vi "Detector Set Config.vi"(8 "error in (no error)":errorcluster, 11 "RIMAS Detector in":refnum<class "RIMAS Detector.lvclass">) -> (0 "error out":errorcluster, 3 "RIMAS Detector out":refnum<class "RIMAS Detector.lvclass">)   [LabVIEW 2022 SP3, in "RIMAS Detector.lvclass"]
uses:
  RIMAS Detector.lvclass
  C:/Development/rimas/RIMAS/Detector/Detector Class/Detector Class.lvclass
  Detector Class.lvclass
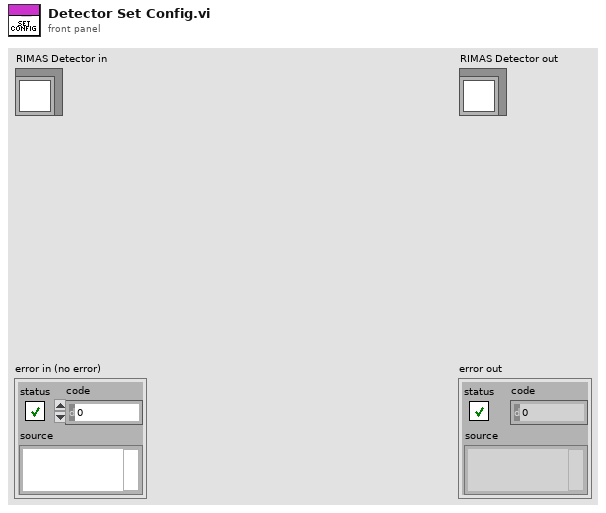
[diagram p1: front panel]
types:
  T1 = typedef "RIMAS Detector Config.ctl" = cluster{"Detector":u16, "Offsets":u16[][], "Detector Computer":T2, "FITS hdr template0":path, "FITS hdr template1":path, "FITS Data File Path":path, "FITS Detector Settings":T3, "Sim Folder":path, "Integration Mode":T4, "Integration Time":dbl, "Frame Int Time":dbl}
  T2 = typedef "RIMAS Detector Server Config.ctl" = cluster{"Machine":string, "Password":string, "FITS File Path":string, "Port":u16, "Header Path":string, "Name":string}
  T3 = typedef "RIMAS Observation Config.ctl" = cluster{"Exp Time Short":dbl, "# of Frames":dbl, "Exp Time Long":dbl, "# of Groups":dbl, "Object Name":string, "Object":string, "Obs Type":string, "Image Type":string, "Observer":string, "Observer Affiliation":string}
  T4 = typedef "Detector enum Detector Integration Mode.ctl" = enum16{"SSR", "CDS", "MEAN", "MEDIAN", "MODE", "MIIN", "MAX"}
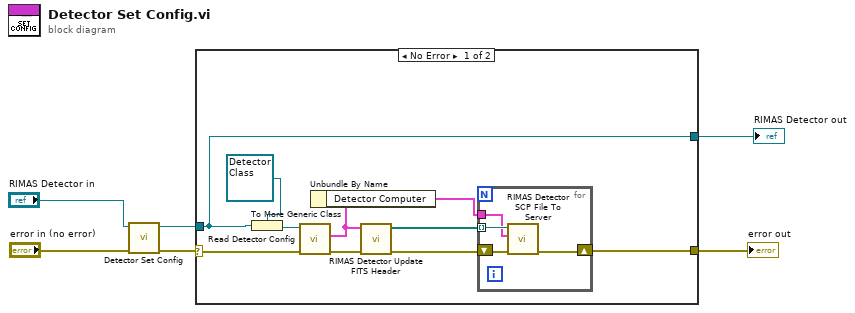
[diagram p0: block diagram]
diagram:
  n1 = call-parent "Detector Set Config.vi"("error in (no error)"="error in (no error)", "Detector Class in"="RIMAS Detector in") -> ("error out"=w3:errorcluster, "Detector Class out"=w4:refnum<class "RIMAS Detector.lvclass">)  [unwired: 8 in]
  n2 = case shown="No Error" w3 {
    selector: w3 -> [w14 w21]
    tunnel: w4 -> [w8 w22]
    tunnel: [w8 w22] -> w2
    tunnel: [w7 w21] -> w1
    frame No Error {
      n3 = To More Generic Class(target class=refnum<class "Detector Class.lvclass"> refnum ("Detector Class.lvclass"), reference=w8) -> (generic class reference=w15:refnum<class "Detector Class.lvclass">)
      n4 = call-dynamic "Read Detector Config.vi"("error in (no error)"=w14, "Detector Class in"=w15) -> ("error out"=w13:errorcluster, "Detector Config"=w11:T1)  [unwired: 7 in, 1 out]
      n5 = Unbundle By Name(w11) -> ("Detector Computer"=w10:T2)
      n6 = call "RIMAS Detector Update FITS Header.vi"("Error In"=w13, "Detector Config"=w11) -> ("Error Out"=w9:errorcluster, "Files"=w12:path[])  [unwired: 8 in]
      n7 = for {
        tunnel: w12 -> [w20] mode=indexing
        tunnel: w10 -> [w19]
        shift-right: [w17] -> w7
        shift-left: w9 -> [w18]
        n8 = call "RIMAS Detector SCP File To Server.vi"("Error In"=w18, "Detector Computer"=w19, "Local File Path"=w20) -> ("Error Out"=w17:errorcluster)  [unwired: 7 in, 1 out]
      }
    }
    frame Error {
    }
  }
  "error out" <- w1
  "RIMAS Detector out" <- w2
